vi "PWM Servo - cRIO.vi"() -> ()   [LabVIEW 2012]
uses:
  <vilib>/rvi/interface/nirviOpenFPGA/nirviOpenFPGA.xnode
  <vilib>/rvi/interface/nirviCloseFPGA/nirviCloseFPGA.xnode
  <vilib>/rvi/interface/nirviReadWriteControl/nirviReadWriteControl.xnode
  C:/Users/dredfern/Documents/robo1/act/2013 ACT Lab_Rev B/Motor Lab A/FPGA Bitfiles/MotorLabAProject_FPGATarget_PWMServoFPGA_HS5lU4NEzhI.lvbitx
  C:/Users/dredfern/Documents/robo1/act/2013 ACT Lab_Rev B/Motor Lab A/PWM Servo FPGA Rev B.vi
  <vilib>/FPGAPlugInAG/Dynamic/niLvFpga_Close_Dynamic.vi
  <vilib>/FPGAPlugInAG/cRIO-9074/niLvFpga_Open_cRIO-9074.vi
  <vilib>/rvi/interface/common/dynamic/niFpgaDynamicAddResources.vi
  NiFpgaLv.dll
  <vilib>/Utility/error.llb/Error Cluster From Error Code.vi
  <vilib>/rvi/interface/Simulation/niFpgaSimulationCallBeginRW.vi
  <vilib>/rvi/errors/niLvFpgaAdjustHostInterfaceError.vi
panel:
  in  "Current PI Gains":T1
  out "Feedback":i16(graph)
  out "Command":i16(graph)
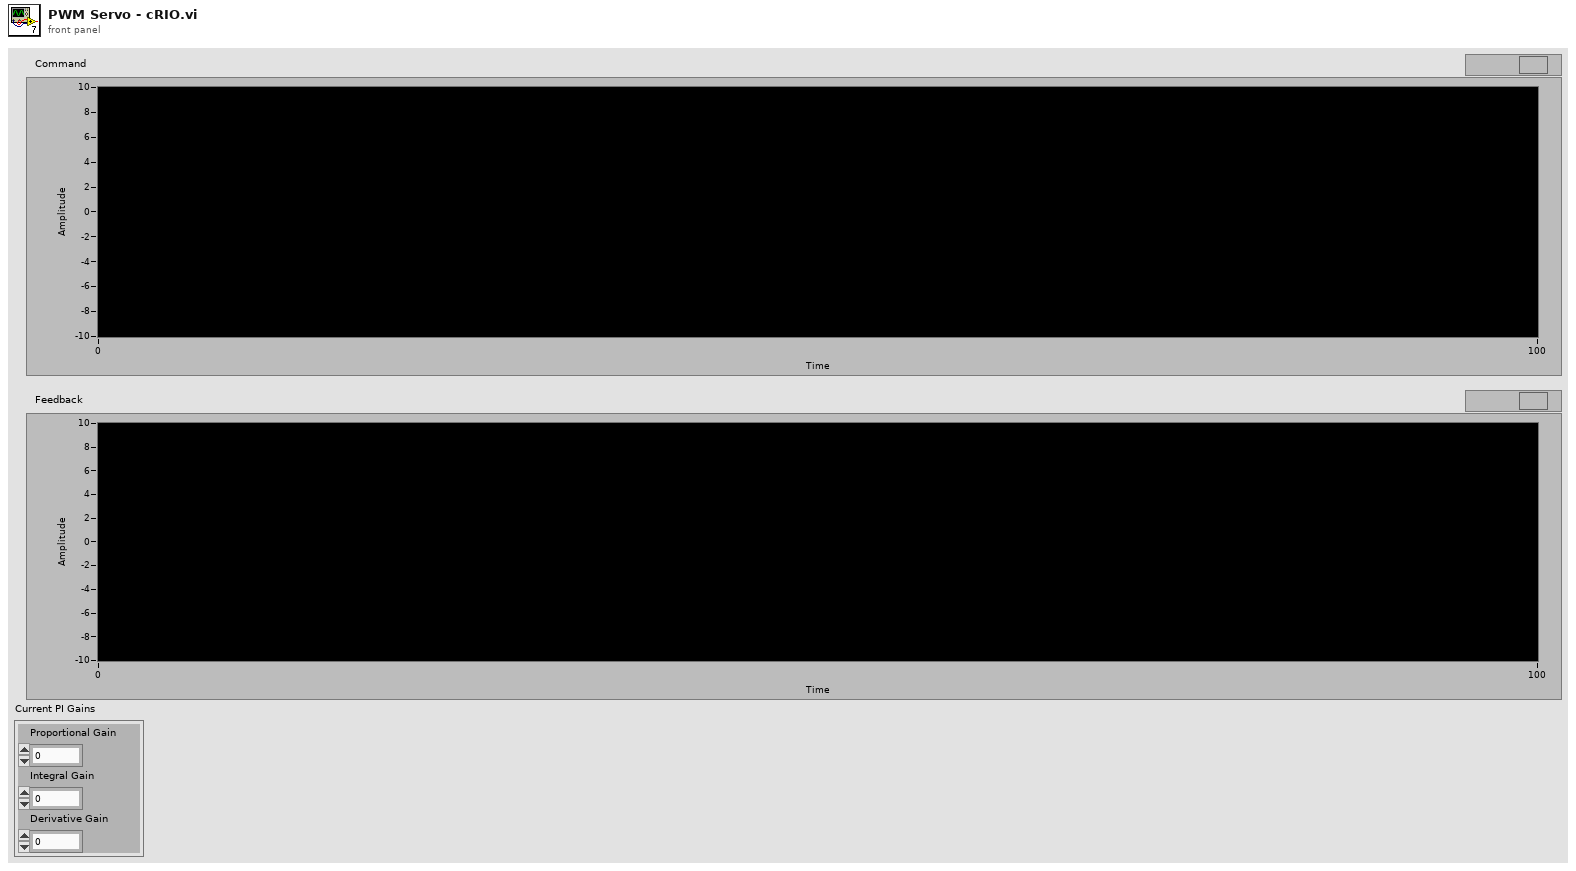
[diagram p1: front panel]
types:
  T1 = cluster{"Proportional Gain":i16, "Integral Gain":i16, "Derivative Gain":i16}
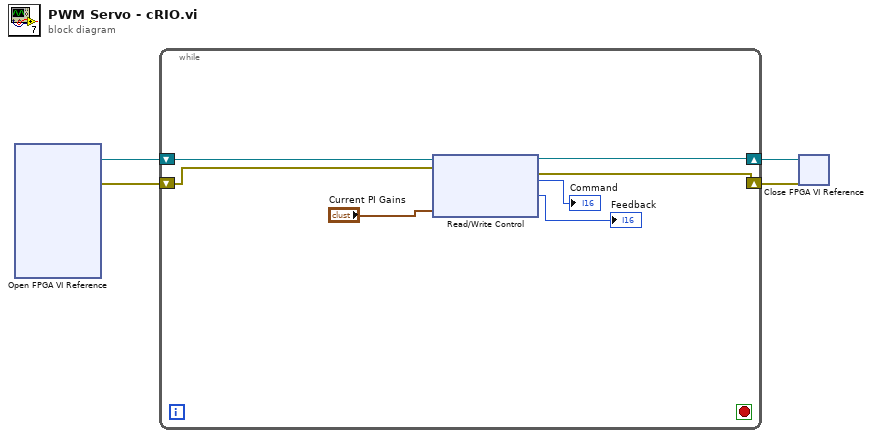
[diagram p0: block diagram]
diagram:
  n1 = xnode "Open FPGA VI Reference"() -> ("FPGA VI Reference Out"=w4:refnum<k20>, "error out"=w3:errorcluster)  [unwired: 2 in]
  n2 = while {
    shift-right: [w9] -> w2
    shift-left: w4 -> [w11]
    shift-right: [w8] -> w1
    shift-left: w3 -> [w10]
    stop <- _ stop-if-true
    n3 = xnode "Read/Write Control"("FPGA VI Reference In"=w11, "error in"=w10, "Current PI Gains"="Current PI Gains") -> ("FPGA VI Reference Out"=w9:refnum<k20>, "error out"=w8:errorcluster, "Current Command"=→"Command":i16, "Current Feedback"=→"Feedback":i16)
  }
  n4 = xnode "Close FPGA VI Reference"("FPGA VI Reference In"=w2, "error in"=w1) -> ()  [unwired: 1 out]
